vi "Test WS Internet Echo.vi"(8 "error in (no error)":errorcluster, 11 "TestCase in":refnum<class "Test Legacy Client.lvclass">) -> (0 "error out":errorcluster, 3 "TestCase out":refnum<class "Test Legacy Client.lvclass">)   [LabVIEW 2013, in "Test Legacy Client.lvclass"]
uses:
  Test Legacy Client.lvclass
  <vilib>/addons/_JKI Toolkits/VI Tester/TestCase.llb/TestCase.lvclass
  WebSockets/WebSockets.lvlib
panel:
  out "Server Headers Out":variant
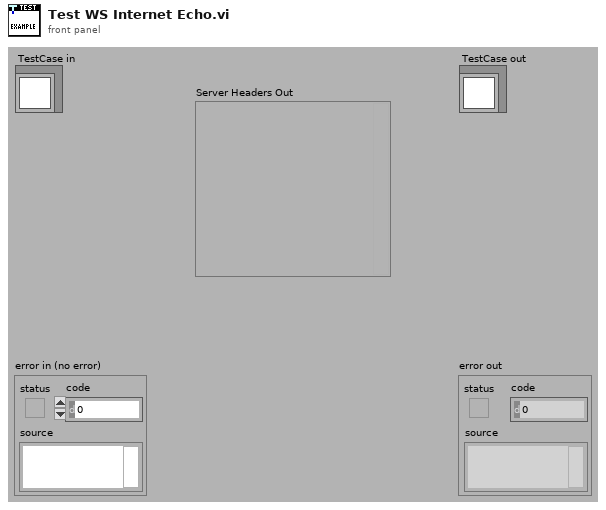
[diagram p1: front panel]
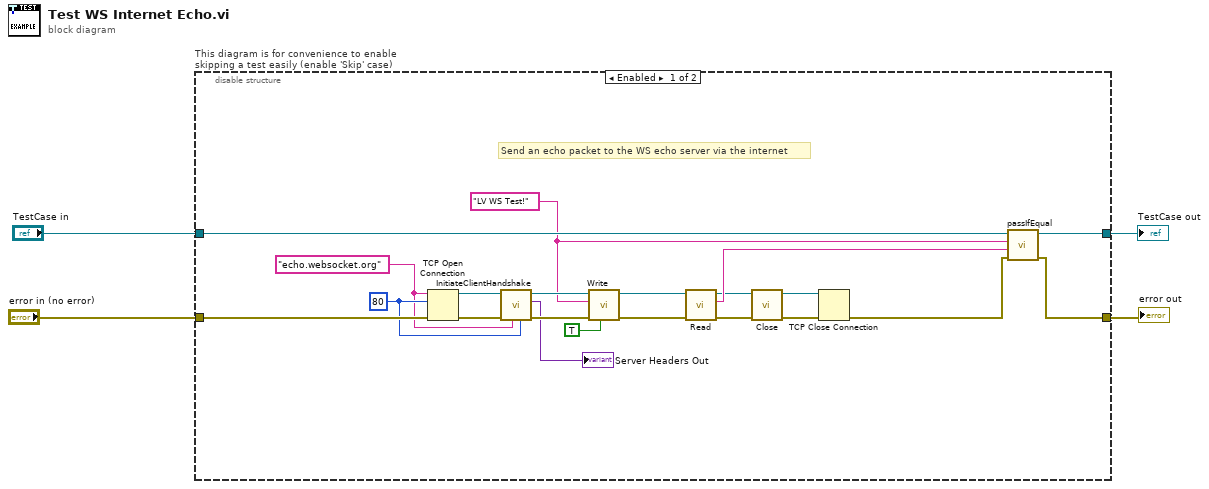
[diagram p0: block diagram]
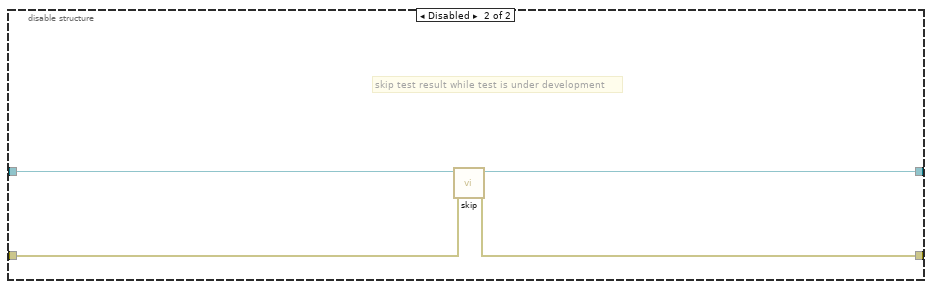
[diagram p2: hidden frame]
diagram:
  n1 = disable-structure "This diagram is for convenience to enable skipping a test easily (enable 'Skip' case)" shown="Enabled" {
    disable-tunnel: "TestCase in" -> [w24 w29]
    disable-tunnel: [w23 w27] -> w1
    disable-tunnel: [w22 w28] -> w3
    disable-tunnel: "error in (no error)" -> [w25 w26]
    frame Enabled {
      w11 = u16 80 ("remote port or service name")
      w5 = "echo.websocket.org" ("address")
      w14 = "LV WS Test!"
      # "Send an echo packet to the WS echo server via the internet"
      n2 = TCP Open Connection(address=w5, remote port or service name=w11, error in (no error)=w25) -> (connection ID=w21:refnum<k5>, error out=w20:errorcluster)  [unwired: 2 in]
      n3 = call "InitiateClientHandshake.vi"("remote port or service name"=w11, "address ('localhost')"=w5, "error in (no error)"=w20, "TCP Connection in"=w21) -> ("error out"=w19:errorcluster, "Server Headers Out"=→"Server Headers Out":variant, "WebSocket Client out"=w18:refnum<class "WebSocket Client.lvclass">)  [unwired: 5 in]
      n4 = call "Write.vi"("Mask payload?"=TRUE, "error in (no error)"=w19, "Data"=w14, "WebSocket in"=w18) -> ("error out"=w17:errorcluster, "WebSocket out"=w16:refnum<class "WebSocket Client.lvclass">)  [unwired: 6 in]
      n5 = call "Read.vi"("error in (no error)"=w17, "WebSocket in"=w16) -> ("error out"=w13:errorcluster, "Data"=w15:string, "WebSocket out"=w9:refnum<class "WebSocket Client.lvclass">)  [unwired: 5 in, 2 out]
      n6 = call "Close.vi"("error in (no error)"=w13, "WebSocket in"=w9) -> ("error out"=w10:errorcluster, "TCP Connection out"=w8:refnum<k5>)  [unwired: 8 in]
      n7 = TCP Close Connection(connection ID=w8, error in (no error)=w10) -> (error out=w12:errorcluster)  [unwired: 1 in, 1 out]
      n8 = call-dynamic "passIfEqual.vi"("error in (no error)"=w12, "y"=w15, "x"=w14, "TestCase in"=w24) -> ("error out"=w22:errorcluster, "TestCase out"=w23:refnum<class "Test Legacy Client.lvclass">)  [unwired: 6 in]
    }
    frame Disabled {
      # "skip test result while test is under development"
      n9 = call <vilib>:"skip.vi"("error in (no error)"=w26, "TestCase in"=w29) -> ("error out"=w28:errorcluster, "TestCase out"=w27:refnum<class "Test Legacy Client.lvclass">)  [unwired: 8 in]
    }
  }
  "error out" <- w3
  "TestCase out" <- w1
